vi "PhysMon-Wait for Next Read.vi"(0 "Hardware Mutex":T1, 5 "Options":T2={"Min Interval"=0.0, "HR from ABR?"=FALSE, "HR Scale"={"Slope"=0.0, "Offset"=0.0, "Limits"={"Min"=0.0, "Max"=0.0}, "term config"=-1}, "Temp Scale"={"Slope"=0.0, "Offset"=0.0, "Limits"={"Min"=0.0, "Max"=0.0}, "term config"=-1}, "Lock?"=FALSE, "Temp Sensor"=enum."YSI", "EKG"={"Sample duration (s)"=0.0}} {"Temp Scale"."term config" items=["default"=-1, "RSE"=10083, "NRSE"=10078, "Differential"=10106, "Pseudodifferential"=12529]; "HR Scale"."term config" items=["default"=-1, "RSE"=10083, "NRSE"=10078, "Differential"=10106, "Pseudodifferential"=12529]}, 11 "Error":errorcluster, 12 "First Call?":bool) -> (4 "Stop?":bool, 8 "Mutex Acquired":bool, 15 "Error Out":errorcluster)   [LabVIEW 2020]
uses:
  Typedefs/PhysMon-Options.ctl
  Typedefs/PhysMon-Scale.ctl
  Typedefs/PhysMon-TempSensor.ctl
  Typedefs/PhysMon-HR From EKG Settings.ctl
  Typedefs/VS-Globals.vi
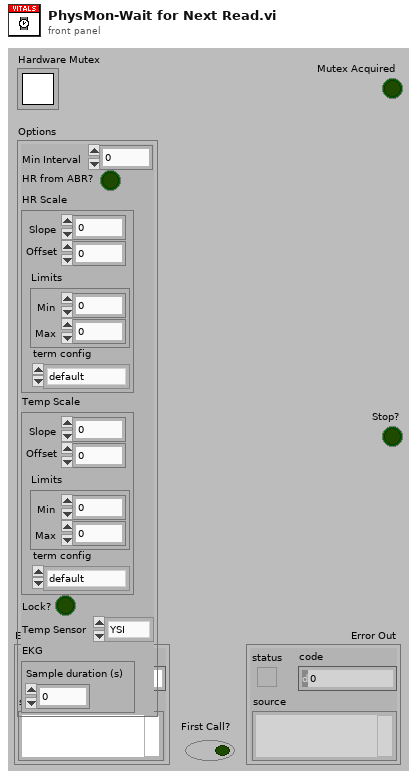
[diagram p1: front panel]
types:
  T1 = typedef "Semaphore RefNum" = refnum<k1>
  T2 = typedef "PhysMon-Options.ctl" = cluster{"Min Interval":dbl, "HR from ABR?":bool, "HR Scale":T3, "Temp Scale":T3, "Lock?":bool, "Temp Sensor":T4, "EKG":T5}
  T3 = typedef "PhysMon-Scale.ctl" = cluster{"Slope":dbl, "Offset":dbl, "Limits":cluster{"Min":dbl, "Max":dbl}, "term config":i32}
  T4 = typedef "PhysMon-TempSensor.ctl" = enum16{"YSI", "FHC", "Custom"}
  T5 = typedef "PhysMon-HR From EKG Settings.ctl" = cluster{"Sample duration (s)":dbl}
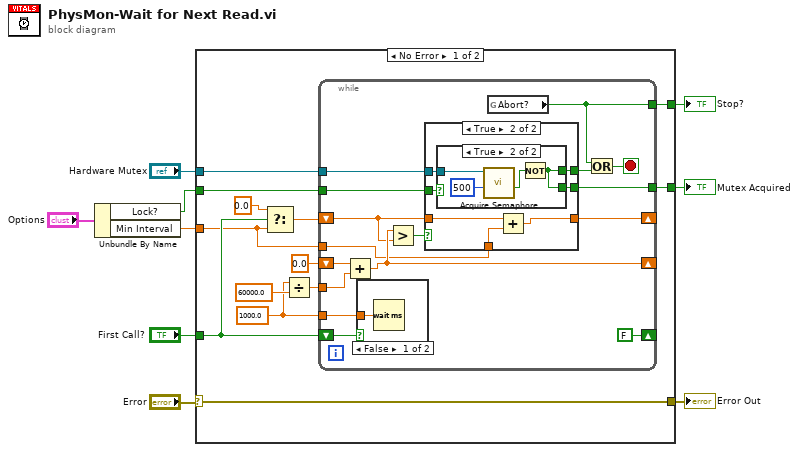
[diagram p0: block diagram]
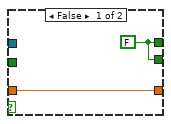
[diagram p3: hidden frame]
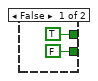
[diagram p4: hidden frame]
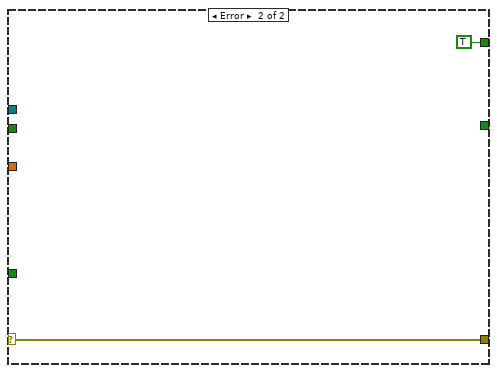
[diagram p5: hidden frame]
diagram:
  n1 = Unbundle By Name("Options") -> ("Lock?"=w2:bool, "Min Interval"=w5:dbl)
  n2 = case shown="No Error" "Error" {
    selector: "Error" -> [w22 w56]
    tunnel: [w22 w56] -> w8
    tunnel: w5 -> [w10 _]
    tunnel: [w12 TRUE ("Abort?")] -> w7
    tunnel: "Hardware Mutex" -> [w17 _]
    tunnel: "First Call?" -> [w14 _]
    tunnel: w2 -> [w13 _]
    tunnel: [w11 _] -> w1
    frame No Error {
      w18 = 1000.0 ("milliseconds to wait")
      n3 = Select(t=0.0 ("f"), s=w14, f=w10) -> (s? t:f=w16:dbl)
      n4 = Divide(x=w18, y=60000.0) -> (x/y=w19:dbl)
      n5 = while {
        tunnel: w18 -> [w37]
        shift-right: [w33] -> _
        shift-left: w16 -> [w34]
        shift-right: [w36] -> _
        shift-left: 0.0 -> [w38]
        tunnel: w19 -> [w31]
        tunnel: w17 -> [w30]
        shift-right: [FALSE ("First call?")] -> _
        shift-left: w14 -> [w29]
        tunnel: w13 -> [w27]
        tunnel: [w26] -> w12
        tunnel: [w24] -> w11
        tunnel: w10 -> [w23]
        stop <- w32 stop-if-true
        n6 = Add(x=w38, y=w31) -> (x+y=w36:dbl)
        n7 = case shown="False" w29 {
          tunnel: w37 -> [w39 _]
          frame False {
            n8 = Wait (ms)(milliseconds to wait=w39) -> ()  [unwired: 1 out]
          }
          frame True {
          }
        }
        n9 = Greater?(x=w36, y=w34) -> (0:w35:bool)
        n10 = case shown="True" w35 {
          tunnel: w34 -> [w41 w48]
          tunnel: [w41 w47] -> w33
          tunnel: [w40 w45] -> w25
          tunnel: w30 -> [_ w46]
          tunnel: w27 -> [_ w44]
          tunnel: [w40 w43] -> w24
          tunnel: w23 -> [_ w42]
          frame False {
            w40 = FALSE
          }
          frame True {
            n11 = case shown="True" w44 {
              tunnel: w46 -> [_ w54]
              tunnel: [TRUE w51] -> w45
              tunnel: [FALSE w51] -> w43
              frame False {
              }
              frame True {
                n12 = call <vilib>:"Acquire Semaphore.vi"("ms timeout (-1)"=500, "semaphore"=w54) -> ("timed out"=w52:bool)  [unwired: 3 in, 2 out]
                n13 = Not(x=w52) -> (.not. x?=w51:bool)
              }
            }
            n14 = Add(x=w48, y=w42) -> (x+y=w47:dbl)
          }
        }
        n15 = global read "VS-Globals.vi" "Abort?"() -> (w26:bool)
        n16 = Or(x=w26, y=w25) -> (x .or. y?=w32:bool)
      }
    }
    frame Error {
    }
  }
  "Error Out" <- w8
  "Stop?" <- w7
  "Mutex Acquired" <- w1
